vi "alert_new.vi"(2 "mode":i32, 3 "error in":errorcluster, 4 "Path":path=path "alert_sound.wav", 5 "Turn on":bool) -> (0 "error out":errorcluster, 1 "appended path":path)   [LabVIEW 2017]
panel:
  in  "device ID":u32 format="%.0x"
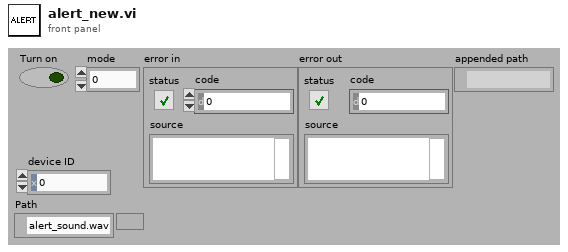
[diagram p1: front panel]
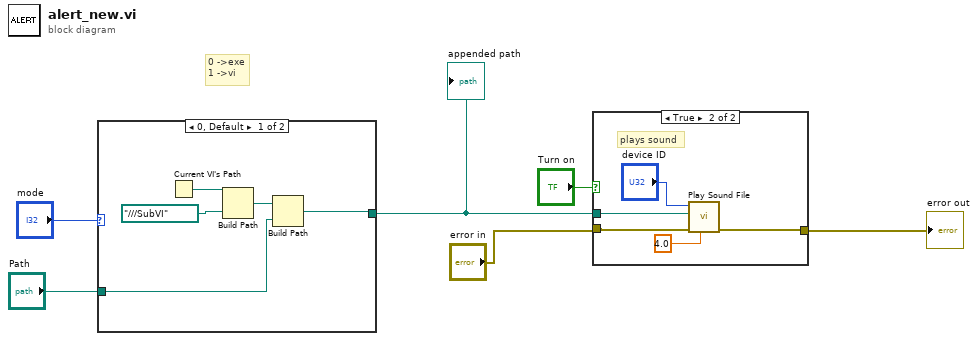
[diagram p0: block diagram]
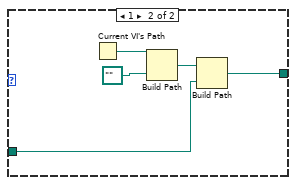
[diagram p2: hidden frame]
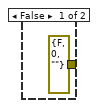
[diagram p3: hidden frame]
diagram:
  # "0 ->exe\n1 ->vi"
  n1 = case shown="0, Default" "mode" {
    tunnel: [w8 w13] -> w4
    tunnel: "Path" -> [w7 w12]
    frame 0, Default {
      n2 = Current VI's Path() -> (path=w11:path)
      n3 = Build Path(base path=w11, name or relative path=path "../../../SubVI") -> (appended path=w9:path)
      n4 = Build Path(base path=w9, name or relative path=w7) -> (appended path=w8:path)
    }
    frame 1 {
      n5 = Current VI's Path() -> (path=w16:path)
      n6 = Build Path(base path=w16, name or relative path=path "..") -> (appended path=w14:path)
      n7 = Build Path(base path=w14, name or relative path=w12) -> (appended path=w13:path)
    }
  }
  "appended path" <- w4
  n8 = case shown="True" "Turn on" {
    tunnel: w4 -> [_ w22]
    tunnel: "error in" -> [_ w21]
    tunnel: [errorcluster {"status"=FALSE, "code"=0, "source"=""} ("error out") w20] -> w5
    frame False {
    }
    frame True {
      # "plays sound"
      n9 = call <vilib>:"Play Sound File.vi"("timeout (sec)"=4.0, "error in (no error)"=w21, "path"=w22, "device ID"="device ID") -> ("error out"=w20:errorcluster)  [unwired: 6 in, 1 out]
    }
  }
  "error out" <- w5
